vi "AddXYGraphCurves.vi"(8 "error in (no error)":errorcluster caption="entrée d'erreur (pas d'erreur)", 9 "CurvIndex":i32, 10 "GraphIndex":i32, 11 "Interface en entrée":refnum<class "Interface.lvclass"> caption="DNL_LabVIEW Object in") -> (0 "error out":errorcluster caption="sortie d'erreur", 2 "IndInGrphCrv":i32, 3 "Interface en sortie":refnum<class "Interface.lvclass"> caption="DNL_LabVIEW Object out")   [LabVIEW 2019, in "Interface.lvclass"]
uses:
  Interface.lvclass
  Interface.lvclass/Interface.ctl
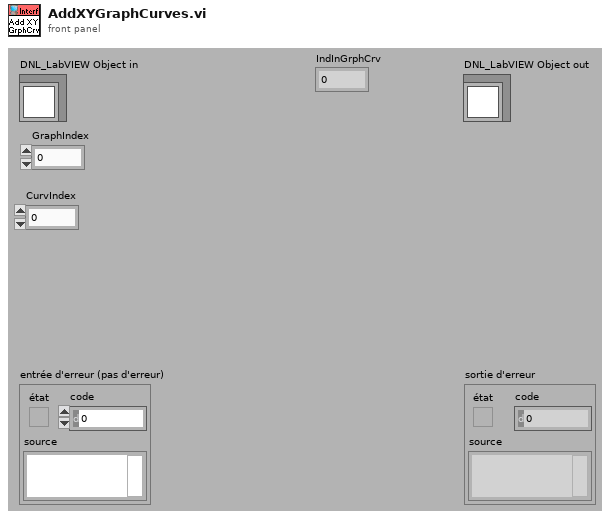
[diagram p1: front panel]
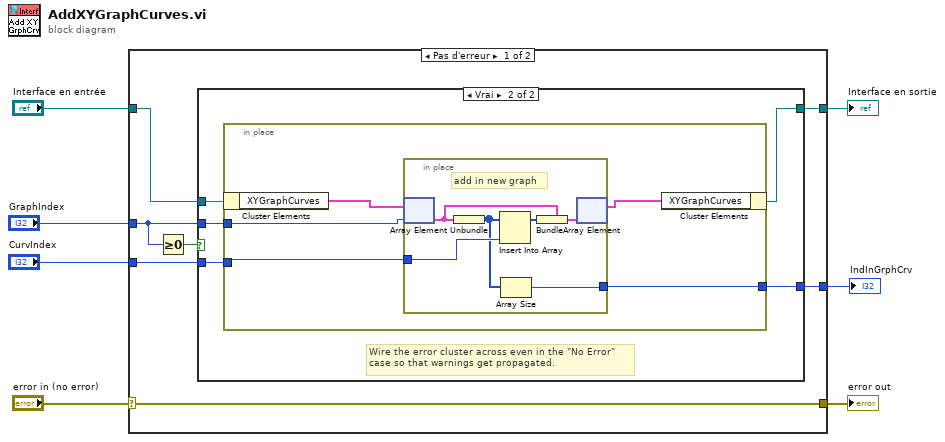
[diagram p0: block diagram]
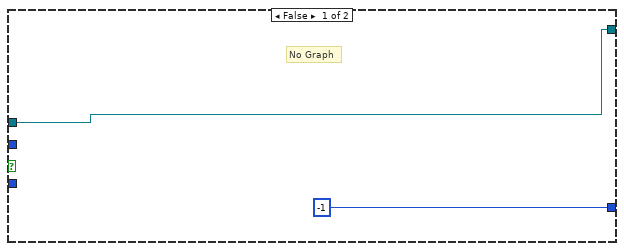
[diagram p2: hidden frame]
diagram:
  n1 = case shown="Pas d'erreur" "error in (no error)" {
    selector: "error in (no error)" -> [w14 w34]
    tunnel: [w14 w34] -> w6
    tunnel: [w11 w33] -> w4
    tunnel: "Interface en entrée" -> [w13 w33]
    tunnel: "CurvIndex" -> [w12 _]
    tunnel: "GraphIndex" -> [w10 _]
    tunnel: [w8 _] -> w1
    frame No Error {
      n2 = Greater Or Equal To 0?(x=w10) -> (x >= 0?=w9:bool)
      n3 = case shown="Vrai" w9 {
        tunnel: w13 -> [w16 w21]
        tunnel: w12 -> [_ w20]
        tunnel: w10 -> [_ w19]
        tunnel: [w16 w18] -> w11
        tunnel: [-1 w17] -> w8
        frame False {
          # "No Graph"
        }
        frame True {
          # "Wire the error cluster across even in the \"No Error\"\ncase so that warnings get propagated."
          n4 = in-place {
            in-place-border: w20 -> [w23]
            in-place-border: w19 -> [w24]
            in-place-border: [w22] -> w17
            n5 = in-place-cluster #1(w21) -> ("XYGraphCurves"=w26:cluster{"Tableau":i32[]}[])
            n6 = in-place {
              in-place-border: w23 -> [w29]
              in-place-border: [w27] -> w22
              # "add in new graph"
              n7 = in-place-array #2(w26, w24) -> (w32:cluster{"Tableau":i32[]})
              n8 = Unbundle(w32) -> ("Tableau"=w28:i32[])
              n9 = Insert Into Array(array=w28, new element=w29) -> (w30:i32[])  [unwired: 1 in]
              n10 = Array Size(array=w28) -> (size(s)=w27:i32)
              n11 = Bundle(cluster=w32, "Tableau"=w30) -> (w31:cluster{"Tableau":i32[]})
              n12 = in-place-array #2(w31) -> (w25:cluster{"Tableau":i32[]}[])  [unwired: 1 out]
            }
            n13 = in-place-cluster #1("XYGraphCurves"=w25) -> (w18:refnum<class "Interface.lvclass">)
          }
        }
      }
    }
    frame Error {
    }
  }
  "error out" <- w6
  "Interface en sortie" <- w4
  "IndInGrphCrv" <- w1
